vi "setResolutionInDigits.vi"(8 "error in (no error)":errorcluster, 10 "Digits":dbl, 11 "DmmNiPxi in":refnum<class "DmmNi.lvclass">) -> (0 "error out":errorcluster, 3 "DmmNiPxi out":refnum<class "DmmNi.lvclass">)   [LabVIEW 2023, in "DmmNi.lvclass"]
doc: "<b>Author:</b> Wolfgang\n<b>Description:</b> set multimeter resolution in digits 4.5, 5.5, 6.5"
uses:
  DmmNi.lvclass
  DmmNi.lvclass/DmmNi.ctl
  Multimeter.lvclass
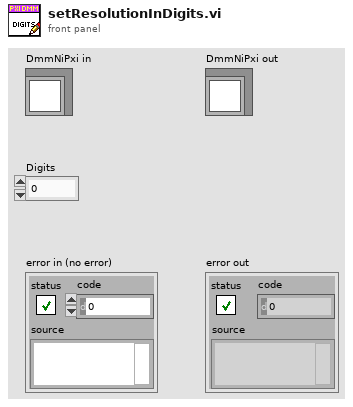
[diagram p1: front panel]
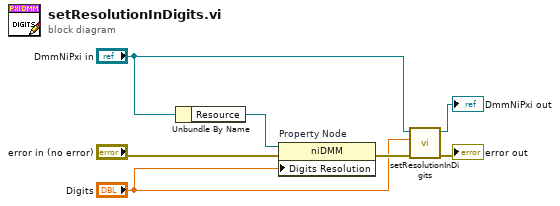
[diagram p0: block diagram]
diagram:
  n1 = Unbundle By Name("DmmNiPxi in") -> ("Resource"=w5:refnum<k15>)
  n2 = property on="Property Node" class="niDMM"(reference=w5, error in="error in (no error)", "Digits Resolution"="Digits") -> (error out=w3:errorcluster)  [unwired: 1 out]
  n3 = call-parent "setResolutionInDigits.vi"("error in (no error)"=w3, "Resolution"="Digits", "Multimeter in"="DmmNiPxi in") -> ("error out"=→"error out":errorcluster, "Multimeter out"=→"DmmNiPxi out":refnum<class "DmmNi.lvclass">)  [unwired: 7 in]
